vi "Low sampling nothing lost.vi"() -> ()   [LabVIEW 2025]
uses:
  <vilib>/Analysis/2dsp.llb/Real FFT.vi
  <vilib>/Analysis/NI_AALBase.lvlib
  <vilib>/Analysis/NI_AALPro.lvlib
panel:
  out "Signals Equal?":bool
  out "The Same Signal":dbl[](graph)
  out "The Same Spectrum":dbl[](graph)
  out "The Spectrum":dbl[](graph)
  out "The Signal":dbl[](graph)
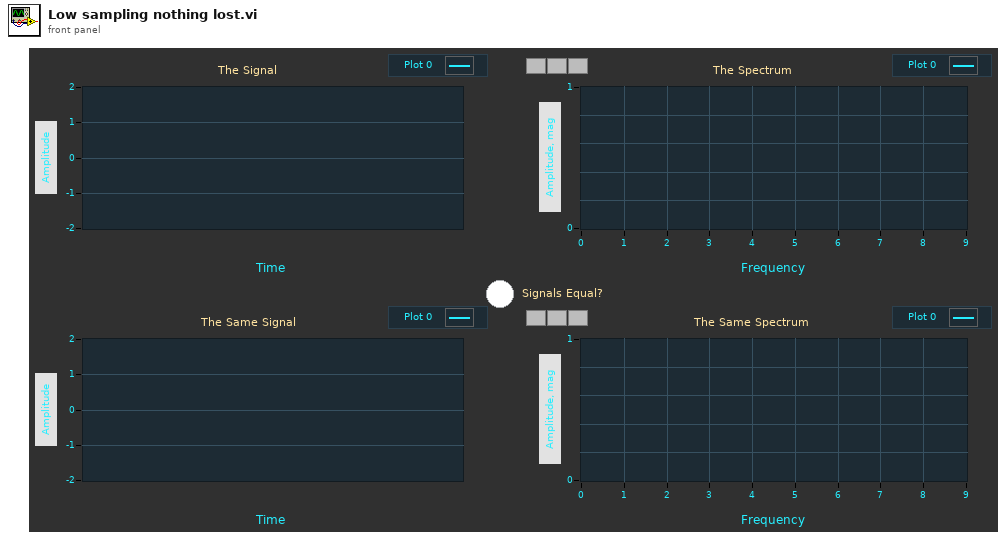
[diagram p1: front panel]
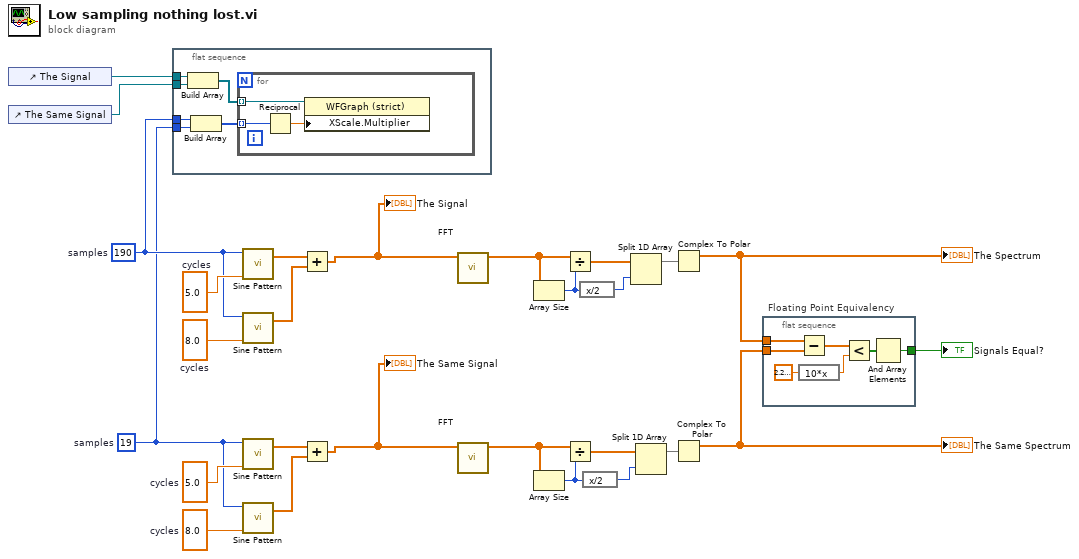
[diagram p0: block diagram]
diagram:
  w19 = 8.0  # cycles
  w20 = 5.0  # cycles
  w1 = 19  # samples
  w22 = 8.0  # cycles
  w21 = 5.0  # cycles
  w2 = 190  # samples
  n1 = control-ref of="The Signal"() -> (w4:refnum<vi>)
  n2 = control-ref of="The Same Signal"() -> (w3:refnum<vi>)
  n3 = flat-sequence {
    tunnel: w4 -> [w33]
    tunnel: w3 -> [w32]
    tunnel: w2 -> [w30]
    tunnel: w1 -> [w29]
    frame #0 {
      n4 = Build Array(w33, w32) -> (w31:refnum<vi>[])
      n5 = Build Array(w30, w29) -> (w28:i32[])
      n6 = for {
        tunnel: w31 -> [w36] mode=indexing
        tunnel: w28 -> [w35] mode=indexing
        n7 = Reciprocal(x=w35) -> (1/x=w34:dbl)
        n8 = property class="WFGraph (strict)"(reference=w36, "XScale.Multiplier"=w34) -> ()  [unwired: 1 in, 2 out]
      }
    }
  }
  n9 = call <vilib>:"Sine Pattern.vi"("cycles"=w21, "samples"=w2) -> ("Sinusoidal Pattern"=w25:dbl[])  [unwired: 2 in, 1 out]
  n10 = call <vilib>:"Sine Pattern.vi"("cycles"=w22, "samples"=w2) -> ("Sinusoidal Pattern"=w23:dbl[])  [unwired: 2 in, 1 out]
  n11 = call <vilib>:"Sine Pattern.vi"("cycles"=w20, "samples"=w1) -> ("Sinusoidal Pattern"=w16:dbl[])  [unwired: 2 in, 1 out]
  n12 = call <vilib>:"Sine Pattern.vi"("cycles"=w19, "samples"=w1) -> ("Sinusoidal Pattern"=w18:dbl[])  [unwired: 2 in, 1 out]
  n13 = Add(x=w25, y=w23) -> (x+y=w24:dbl[])
  "The Signal" <- w24
  n14 = Add(x=w16, y=w18) -> (x+y=w17:dbl[])
  "The Same Signal" <- w17
  n15 = call-poly <vilib>:"FFT.vi"("X"=w24) -> ("FFT {X}"=w27:cdb[])  [unwired: 9 in, 1 out]
  n16 = call-poly <vilib>:"FFT.vi"("X"=w17) -> ("FFT {X}"=w14:cdb[])  [unwired: 9 in, 1 out]
  n17 = Array Size(array=w27) -> (size(s)=w9:i32)
  n18 = Array Size(array=w14) -> (size(s)=w10:i32)
  n19 = Divide(x=w27, y=w9) -> (x/y=w26:cdb[])
  n20 = Divide(x=w14, y=w10) -> (x/y=w15:cdb[])
  n21 = expression code="x/2"(w9) -> (w7:i32)
  n22 = expression code="x/2"(w10) -> (w8:i32)
  n23 = Split 1D Array(array=w26, index=w7) -> (first subarray=w12:cdb[])  [unwired: 1 out]
  n24 = Split 1D Array(array=w15, index=w8) -> (first subarray=w11:cdb[])  [unwired: 1 out]
  n25 = Complex To Polar(r * e^(i*theta)=w12) -> (r=w6:dbl[])  [unwired: 1 out]
  "The Spectrum" <- w6
  n26 = Complex To Polar(r * e^(i*theta)=w11) -> (r=w5:dbl[])  [unwired: 1 out]
  "The Same Spectrum" <- w5
  n27 = flat-sequence "Floating Point Equivalency" {
    tunnel: [w43] -> w13
    tunnel: w6 -> [w39]
    tunnel: w5 -> [w38]
    frame #0 {
      n28 = Subtract(x=w39, y=w38) -> (x-y=w42:dbl[])
      n29 = expression code="10*x"(2.220446049250313e-16) -> (w37:dbl)
      n30 = Less?(x=w42, y=w37) -> (x < y?=w41:bool[])
      n31 = And Array Elements(Boolean array=w41) -> (logical AND=w43:bool)
    }
  }
  "Signals Equal?" <- w13
